vi "Read Scalar Data.vi"(8 "error in (no error)":errorcluster, 10 "Values":dbl[](array[numeric]), 11 "Cluster":T1 {"Data Type" format="%.0x"}) -> (0 "error out":errorcluster, 2 "Values":dbl[](array[numeric]), 3 "Cluster":T1 {"Data Type" format="%.0x"})   [LabVIEW 2016, in "FPGA Addon Engine.lvlib"]
uses:
  FPGA Addon Engine.lvlib
  Types/Register Settings.ctl
  FPGA-Resource-Manager-APIs/Source/Shared/Types/Data Type.ctl
  FPGA-Resource-Manager-APIs/Source/Shared/Types/Scalar Type.ctl
  <vilib>/rvi/errors/niLvFpgaAdjustHostInterfaceError.vi
  <vilib>/Utility/error.llb/Error Cluster From Error Code.vi
  <vilib>/rvi/interface/nirviReadWriteControl/nirviReadWriteControl.xnode
  NiFpgaLv.dll
  <vilib>/rvi/interface/Simulation/niFpgaSimulationCallBeginRW.vi
  FPGA-Resource-Manager-APIs/Source/Shared/FPGA RM Shared API.lvlib
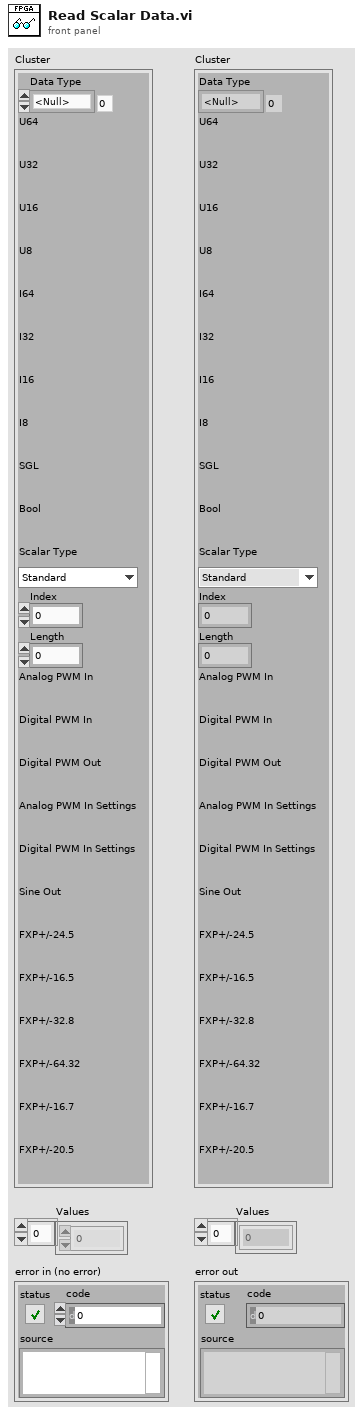
[diagram p1: front panel]
types:
  T1 = typedef "FPGA Addon Engine.lvlib/Register Settings.ctl" = cluster{"Data Type":T2, "U64":refnum<k20>, "U32":refnum<k20>, "U16":refnum<k20>, "U8":refnum<k20>, "I64":refnum<k20>, "I32":refnum<k20>, "I16":refnum<k20>, "I8":refnum<k20>, "SGL":refnum<k20>, "Bool":refnum<k20>, "Scalar Type":T3, "Index":i32, "Length":i32, "Analog PWM In":refnum<k20>, "Digital PWM In":refnum<k20>, "Digital PWM Out":refnum<k20>, "Analog PWM In Settings":refnum<k20>, "Digital PWM In Settings":refnum<k20>, "Sine Out":refnum<k20>, "FXP+/-24.5":refnum<k20>, "FXP+/-16.5":refnum<k20>, "FXP+/-32.8":refnum<k20>, "FXP+/-64.32":refnum<k20>, "FXP+/-16.7":refnum<k20>, "FXP+/-20.5":refnum<k20>}
  T2 = typedef "FPGA RM Shared API.lvlib/Data Type.ctl" = enum8{"<Null>", "I8", "I16", "I32", "I64", "U8", "U16", "U32", "U64", "SGL", "Boolean", "Analog PWM In Settings", "Analog PWM In", "Digital PWM In Settings", "Digital PWM In", "Digital PWM Out", "Sine Out", "FXP+/-24.5", "FXP+/-16.5", "FXP+/-32.8", "FXP+/-64.32", "FXP+/-16.7", "FXP+/-20.5"}
  T3 = typedef "FPGA RM Shared API.lvlib/Scalar Type.ctl" = enum16{"Standard", "Bitpacked"}
  T4 = cluster{"ACTIVE TICKS":u32, "INACTIVE TICKS":u32, "ACQ TICKS":u32, "ACTIVE VOLTAGE":fxp<+/-,32,8>, "INACTIVE VOLTAGE":fxp<+/-,32,8>}
  T5 = cluster{"ACTIVE TICKS":u32, "INACTIVE TICKS":u32, "ACQ TICKS":u32}
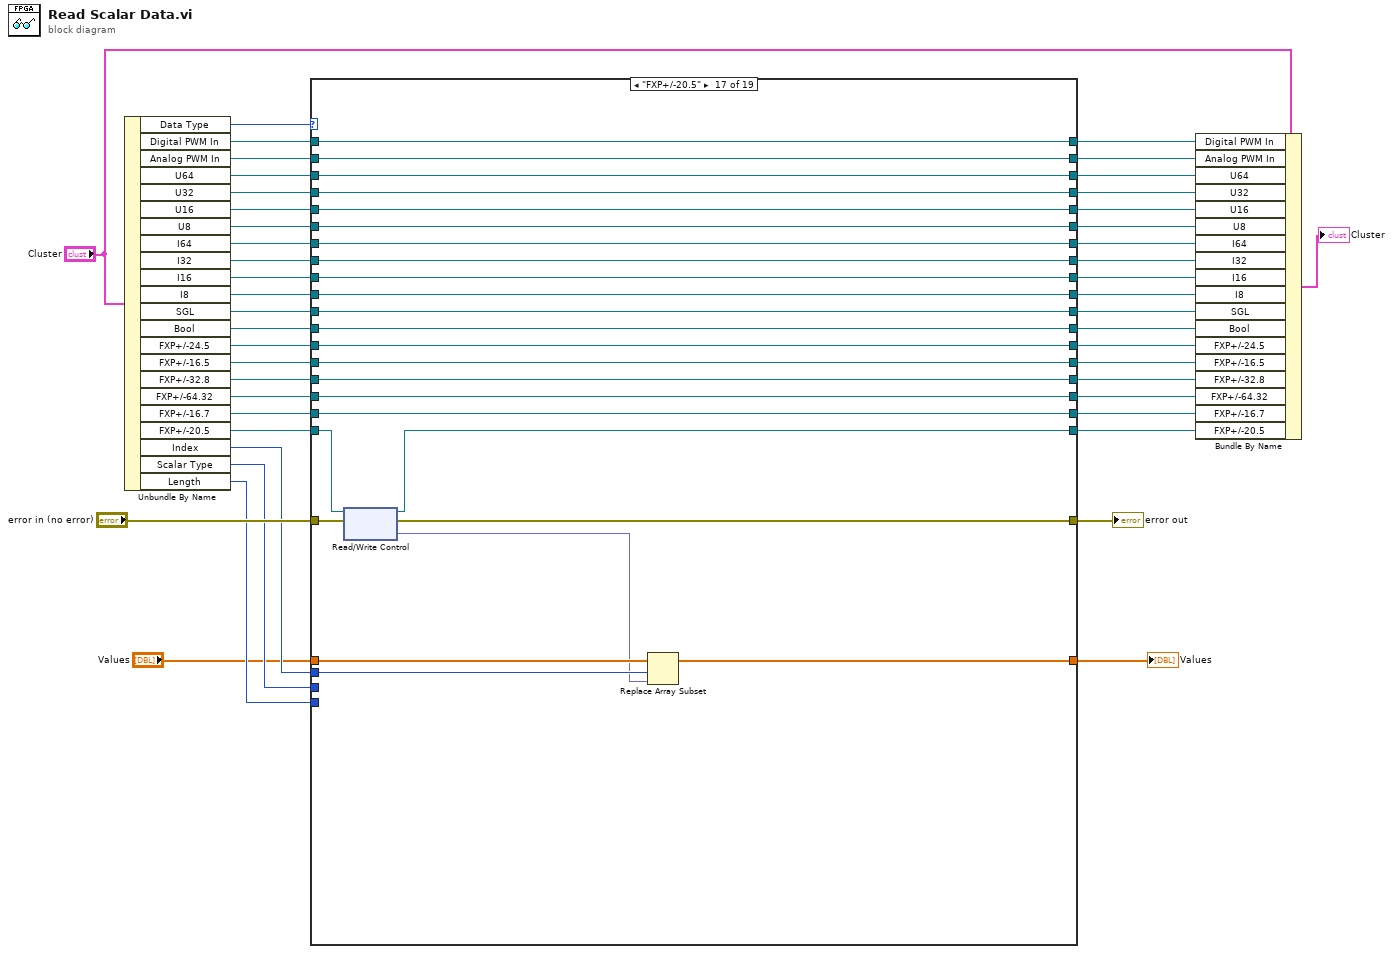
[diagram p0: block diagram]
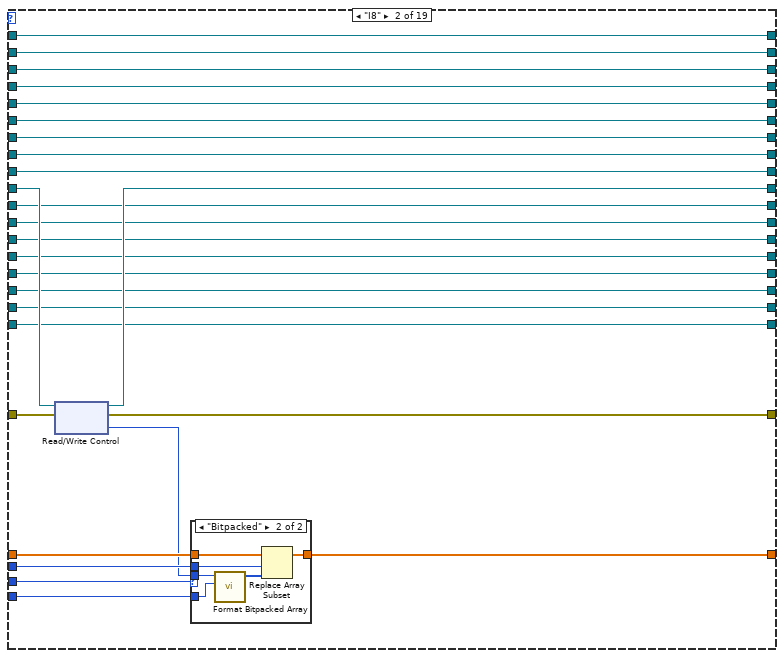
[diagram p3: hidden frame]
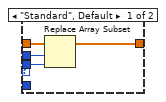
[diagram p4: hidden frame]
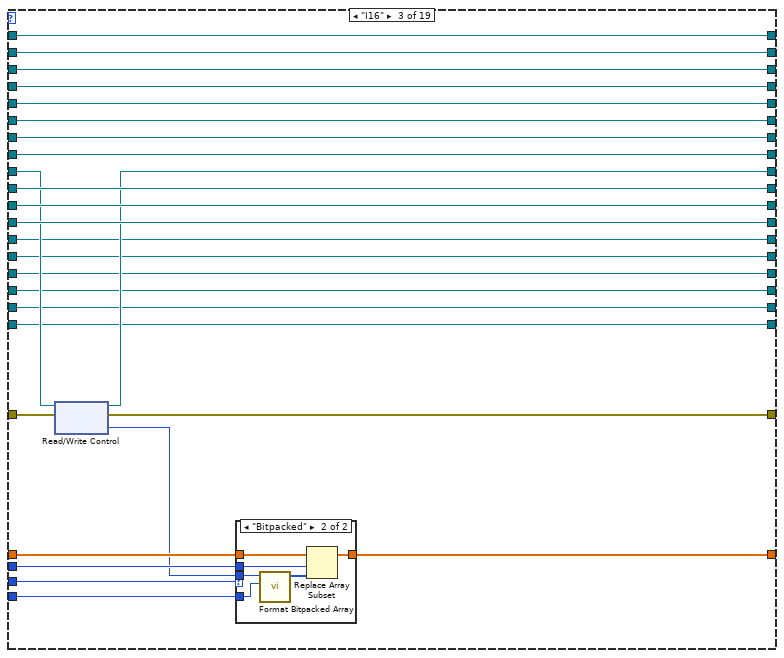
[diagram p5: hidden frame]
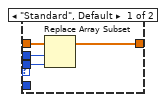
[diagram p6: hidden frame]
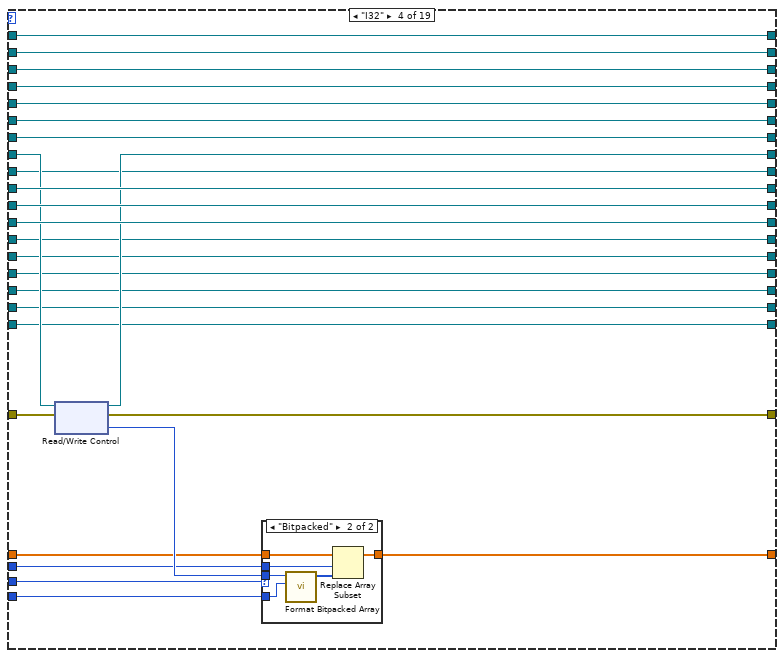
[diagram p7: hidden frame]
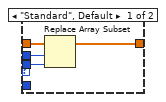
[diagram p8: hidden frame]
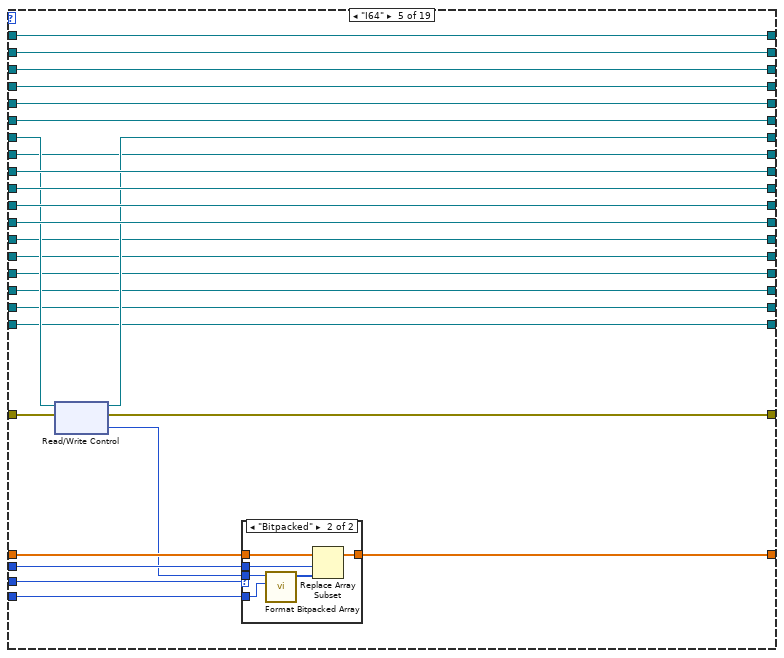
[diagram p9: hidden frame]
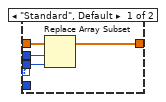
[diagram p10: hidden frame]
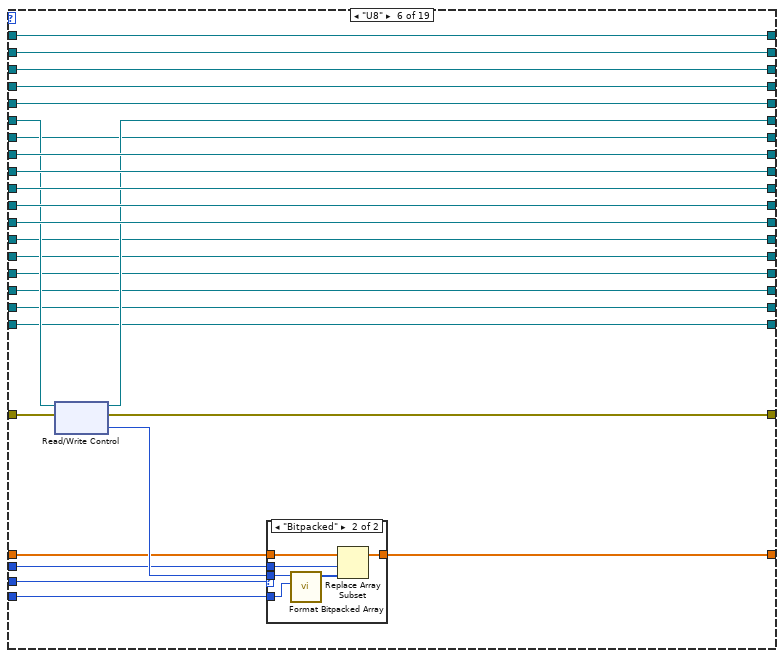
[diagram p11: hidden frame]
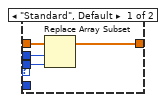
[diagram p12: hidden frame]
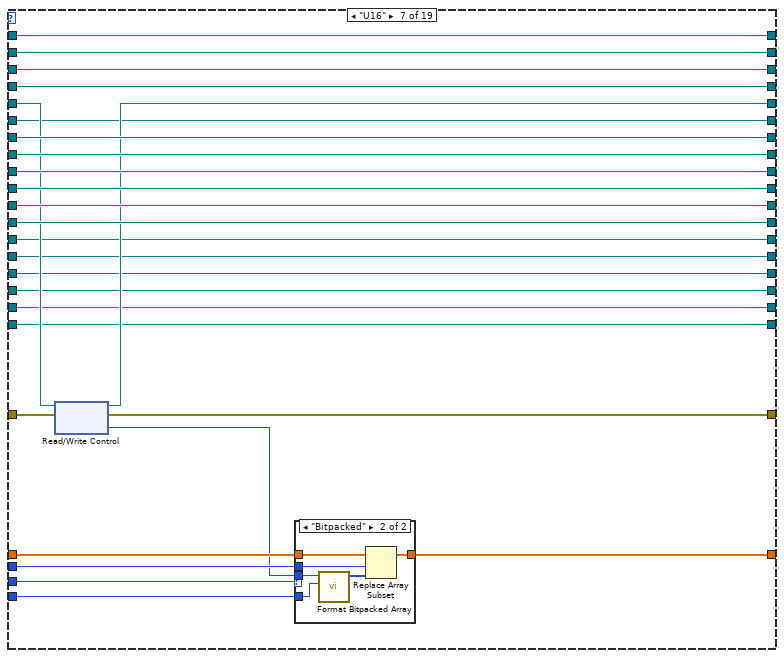
[diagram p13: hidden frame]
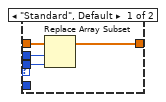
[diagram p14: hidden frame]
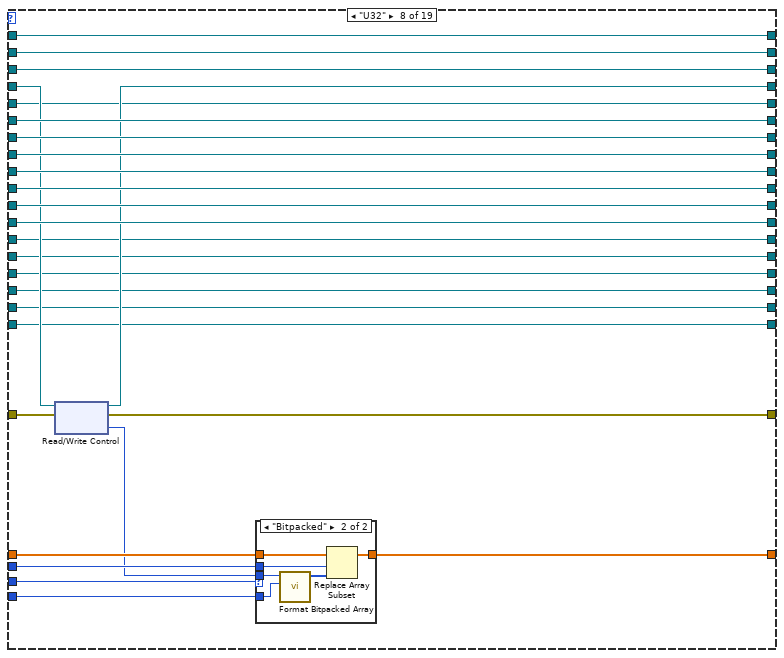
[diagram p15: hidden frame]
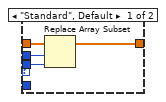
[diagram p16: hidden frame]
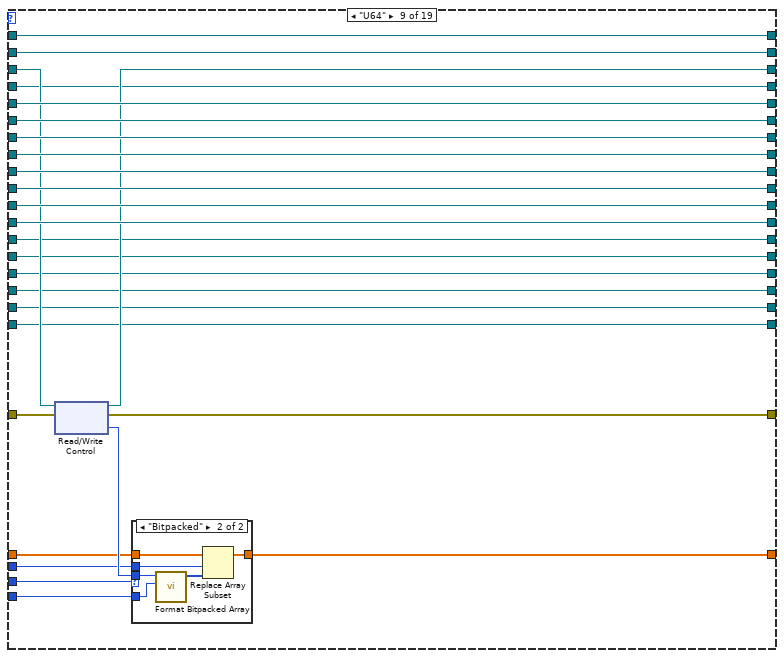
[diagram p17: hidden frame]
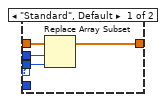
[diagram p18: hidden frame]
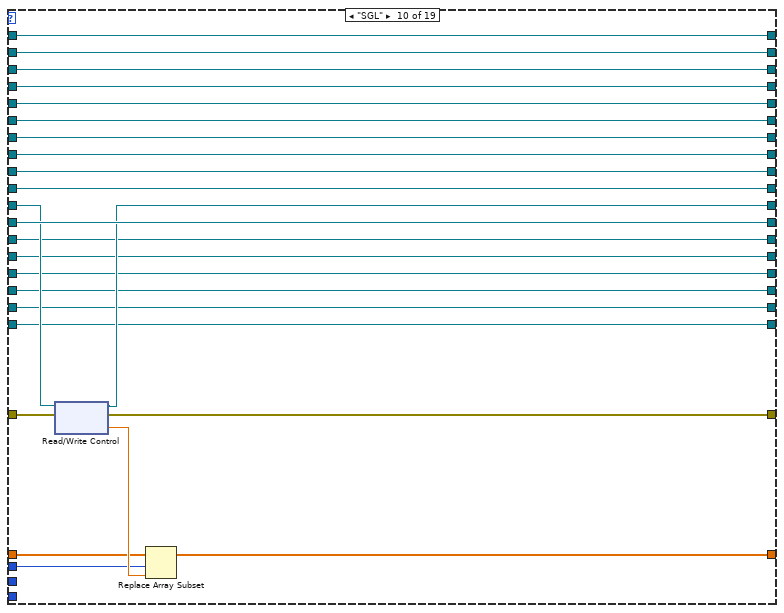
[diagram p19: hidden frame]
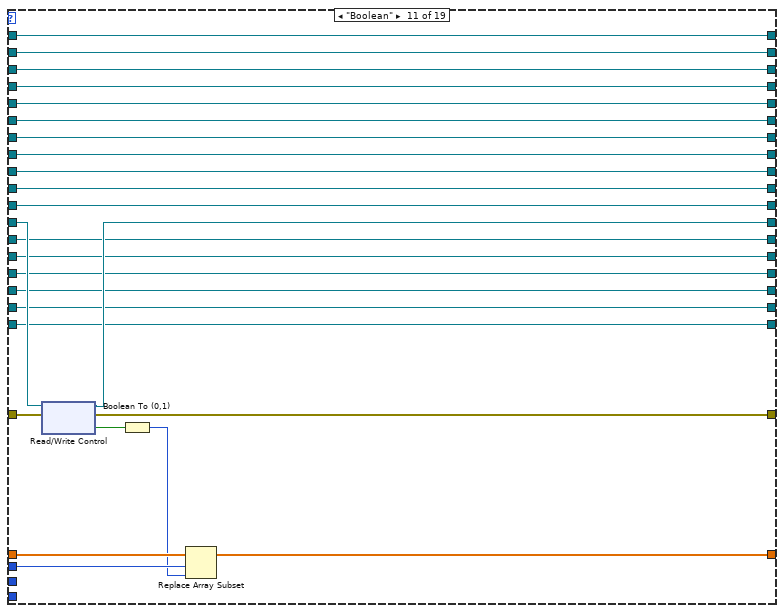
[diagram p20: hidden frame]
diagram:
  n1 = Unbundle By Name("Cluster") -> ("Data Type"=w46:T2, "Digital PWM In"=w14:refnum<k20>, "Analog PWM In"=w15:refnum<k20>, "U64"=w23:refnum<k20>, "U32"=w25:refnum<k20>, "U16"=w27:refnum<k20>, "U8"=w29:refnum<k20>, "I64"=w31:refnum<k20>, "I32"=w33:refnum<k20>, "I16"=w35:refnum<k20>, "I8"=w45:refnum<k20>, "SGL"=w39:refnum<k20>, "Bool"=w38:refnum<k20>, "FXP+/-24.5"=w12:refnum<k20>, "FXP+/-16.5"=w9:refnum<k20>, "FXP+/-32.8"=w8:refnum<k20>, "FXP+/-64.32"=w5:refnum<k20>, "FXP+/-16.7"=w3:refnum<k20>, "FXP+/-20.5"=w1:refnum<k20>, "Index"=w19:i32, "Scalar Type"=w20:T3, "Length"=w21:i32)
  n2 = case shown="\"FXP+/-20.5\"" w46 {
    tunnel: w45 -> [w64 w93 w120 w158 w196 w234 w272 w310 w348 w384 w411 w436 w461 w486 w511 w536 w561 w601 w651]
    tunnel: "error in (no error)" -> [w56 w92 w130 w167 w204 w241 w278 w315 w352 w387 w413 w438 w463 w488 w513 w538 w563 w598 w648]
    tunnel: [w56 w91 w129 w166 w203 w240 w277 w314 w351 w386 w412 w437 w462 w487 w512 w537 w562 w597 w647] -> w43
    tunnel: [w64 w90 w120 w158 w196 w234 w272 w310 w348 w384 w411 w436 w461 w486 w511 w536 w561 w601 w651] -> w41
    tunnel: [w65 w89 w128 w165 w202 w239 w276 w313 w350 w375 w401 w428 w453 w478 w503 w528 w553 w600 w650] -> w40
    tunnel: w39 -> [w65 w89 w128 w165 w202 w239 w276 w313 w350 w377 w401 w428 w453 w478 w503 w528 w553 w600 w650]
    tunnel: w38 -> [w66 w88 w127 w164 w201 w238 w275 w312 w349 w385 w403 w421 w447 w472 w497 w522 w547 w599 w649]
    tunnel: [w66 w88 w127 w164 w201 w238 w275 w312 w349 w385 w402 w421 w447 w472 w497 w522 w547 w599 w649] -> w37
    tunnel: [w63 w87 w118 w155 w195 w233 w271 w309 w347 w383 w410 w435 w460 w485 w510 w535 w560 w602 w652] -> w36
    tunnel: w35 -> [w63 w87 w119 w155 w195 w233 w271 w309 w347 w383 w410 w435 w460 w485 w510 w535 w560 w602 w652]
    tunnel: [w62 w86 w126 w156 w192 w232 w270 w308 w346 w382 w409 w434 w459 w484 w509 w534 w559 w603 w653] -> w34
    tunnel: w33 -> [w62 w86 w126 w157 w192 w232 w270 w308 w346 w382 w409 w434 w459 w484 w509 w534 w559 w603 w653]
    tunnel: [w61 w85 w125 w163 w193 w229 w269 w307 w345 w381 w408 w433 w458 w483 w508 w533 w558 w604 w654] -> w32
    tunnel: w31 -> [w61 w85 w125 w163 w194 w229 w269 w307 w345 w381 w408 w433 w458 w483 w508 w533 w558 w604 w654]
    tunnel: [w60 w84 w124 w162 w200 w230 w266 w306 w344 w380 w407 w432 w457 w482 w507 w532 w557 w605 w655] -> w30
    tunnel: w29 -> [w60 w84 w124 w162 w200 w231 w266 w306 w344 w380 w407 w432 w457 w482 w507 w532 w557 w605 w655]
    tunnel: [w59 w83 w123 w161 w199 w237 w267 w303 w343 w379 w406 w431 w456 w481 w506 w531 w556 w606 w656] -> w28
    tunnel: w27 -> [w59 w83 w123 w161 w199 w237 w268 w303 w343 w379 w406 w431 w456 w481 w506 w531 w556 w606 w656]
    tunnel: [w58 w82 w122 w160 w198 w236 w274 w304 w340 w378 w405 w430 w455 w480 w505 w530 w555 w607 w657] -> w26
    tunnel: w25 -> [w58 w82 w122 w160 w198 w236 w274 w305 w340 w378 w405 w430 w455 w480 w505 w530 w555 w607 w657]
    tunnel: [w57 w81 w121 w159 w197 w235 w273 w311 w341 w376 w404 w429 w454 w479 w504 w529 w554 w608 w658] -> w24
    tunnel: w23 -> [w57 w81 w121 w159 w197 w235 w273 w311 w342 w376 w404 w429 w454 w479 w504 w529 w554 w608 w658]
    tunnel: w21 -> [_ w77 w114 w149 w188 w225 w265 w298 w336 _ _ _ _ _ _ _ _ _ _]
    tunnel: w20 -> [_ w78 w115 w150 w189 w224 w264 w299 w337 _ _ _ _ _ _ _ _ _ _]
    tunnel: w19 -> [_ w79 w116 w153 w190 w226 w263 w300 w338 w373 w399 w427 w452 w477 w502 w527 w552 w580 w630]
    tunnel: "Values" -> [w55 w80 w117 w152 w191 w227 w262 w302 w335 w372 w398 w426 w451 w476 w501 w526 w551 w582 w632]
    tunnel: [w55 w75 w112 w151 w186 w223 w261 w301 w334 w371 w396 w425 w450 w475 w500 w525 w550 w581 w631] -> w17
    tunnel: [w54 w73 w110 w147 w184 w221 w258 w295 w332 w369 w394 w423 w448 w473 w498 w523 w548 w595 w628] -> w16
    tunnel: w15 -> [w54 w73 w110 w147 w184 w221 w258 w295 w332 w369 w394 w423 w448 w473 w498 w523 w548 w596 w628]
    tunnel: w14 -> [w53 w74 w111 w148 w185 w222 w259 w296 w333 w370 w395 w424 w449 w474 w499 w524 w549 w609 w627]
    tunnel: [w53 w74 w111 w148 w185 w222 w259 w296 w333 w370 w395 w424 w449 w474 w499 w524 w549 w609 w626] -> w13
    tunnel: w12 -> [w52 w72 w109 w146 w183 w220 w257 w294 w331 w368 w393 w422 w441 w469 w495 w520 w545 w569 w620]
    tunnel: [w52 w72 w109 w146 w183 w220 w257 w294 w331 w368 w393 w420 w441 w469 w495 w520 w545 w569 w620] -> w11
    tunnel: [w51 w71 w108 w145 w182 w219 w256 w293 w330 w367 w392 w418 w442 w468 w494 w519 w544 w568 w619] -> w10
    tunnel: w9 -> [w51 w71 w108 w145 w182 w219 w256 w293 w330 w367 w392 w418 w443 w468 w494 w519 w544 w568 w619]
    tunnel: w8 -> [w50 w70 w107 w144 w181 w218 w255 w292 w329 w366 w391 w417 w445 w467 w493 w518 w543 w567 w618]
    tunnel: [w50 w70 w107 w144 w181 w218 w255 w292 w329 w366 w391 w417 w445 w466 w493 w518 w543 w567 w618] -> w7
    tunnel: [w49 w69 w106 w143 w180 w217 w254 w291 w328 w365 w390 w416 w444 w470 w491 w517 w542 w566 w617] -> w6
    tunnel: w5 -> [w49 w69 w106 w143 w180 w217 w254 w291 w328 w365 w390 w416 w444 w470 w492 w517 w542 w566 w617]
    tunnel: [w48 w68 w105 w142 w179 w216 w253 w290 w327 w364 w389 w415 w440 w465 w490 w515 w539 w565 w616] -> w4
    tunnel: w3 -> [w48 w68 w105 w142 w179 w216 w253 w290 w327 w364 w389 w415 w440 w465 w490 w516 w539 w565 w616]
    tunnel: [w47 w67 w104 w141 w178 w215 w252 w289 w326 w363 w388 w414 w439 w464 w489 w514 w541 w564 w615] -> w2
    tunnel: w1 -> [w47 w67 w104 w141 w178 w215 w252 w289 w326 w363 w388 w414 w439 w464 w489 w514 w540 w564 w615]
    frame "<Null>", Default {
    }
    frame "I8" {
      n3 = xnode "Read/Write Control"("FPGA VI Reference In"=w93, "error in"=w92) -> ("FPGA VI Reference Out"=w90:refnum<k20>, "error out"=w91:errorcluster, "Value"=w76:i8)
      n4 = case shown="\"Bitpacked\"" w78 {
        tunnel: w80 -> [w97 w101]
        tunnel: [w96 w100] -> w75
        tunnel: w76 -> [w95 w103]
        tunnel: w79 -> [w94 w98]
        tunnel: w77 -> [_ w102]
        frame "Standard", Default {
          n5 = Replace Array Subset(array=w97, new element=w95, index=w94) -> (w96:dbl[])
        }
        frame "Bitpacked" {
          n6 = call "Format Bitpacked Array.vi"("Length"=w102, "Value"=w103) -> ("Array"=w99:i16[])  [unwired: 9 in]
          n7 = Replace Array Subset(array=w101, new element=w99, index=w98) -> (w100:dbl[])
        }
      }
    }
    frame "I16" {
      n8 = xnode "Read/Write Control"("FPGA VI Reference In"=w119, "error in"=w130) -> ("FPGA VI Reference Out"=w118:refnum<k20>, "error out"=w129:errorcluster, "Value"=w113:i16)
      n9 = case shown="\"Bitpacked\"" w115 {
        tunnel: w117 -> [w134 w138]
        tunnel: [w133 w137] -> w112
        tunnel: w113 -> [w132 w140]
        tunnel: w116 -> [w131 w135]
        tunnel: w114 -> [_ w139]
        frame "Standard", Default {
          n10 = Replace Array Subset(array=w134, new element=w132, index=w131) -> (w133:dbl[])
        }
        frame "Bitpacked" {
          n11 = call "Format Bitpacked Array.vi"("Length"=w139, "Value"=w140) -> ("Array"=w136:i16[])  [unwired: 9 in]
          n12 = Replace Array Subset(array=w138, new element=w136, index=w135) -> (w137:dbl[])
        }
      }
    }
    frame "I32" {
      n13 = xnode "Read/Write Control"("FPGA VI Reference In"=w157, "error in"=w167) -> ("FPGA VI Reference Out"=w156:refnum<k20>, "error out"=w166:errorcluster, "Value"=w154:i32)
      n14 = case shown="\"Bitpacked\"" w150 {
        tunnel: w152 -> [w171 w175]
        tunnel: [w170 w174] -> w151
        tunnel: w154 -> [w169 w177]
        tunnel: w153 -> [w168 w172]
        tunnel: w149 -> [_ w176]
        frame "Standard", Default {
          n15 = Replace Array Subset(array=w171, new element=w169, index=w168) -> (w170:dbl[])
        }
        frame "Bitpacked" {
          n16 = call "Format Bitpacked Array.vi"("Length"=w176, "Value"=w177) -> ("Array"=w173:i16[])  [unwired: 9 in]
          n17 = Replace Array Subset(array=w175, new element=w173, index=w172) -> (w174:dbl[])
        }
      }
    }
    frame "I64" {
      n18 = xnode "Read/Write Control"("FPGA VI Reference In"=w194, "error in"=w204) -> ("FPGA VI Reference Out"=w193:refnum<k20>, "error out"=w203:errorcluster, "Value"=w187:i64)
      n19 = case shown="\"Bitpacked\"" w189 {
        tunnel: w191 -> [w208 w212]
        tunnel: [w207 w211] -> w186
        tunnel: w187 -> [w206 w214]
        tunnel: w190 -> [w205 w209]
        tunnel: w188 -> [_ w213]
        frame "Standard", Default {
          n20 = Replace Array Subset(array=w208, new element=w206, index=w205) -> (w207:dbl[])
        }
        frame "Bitpacked" {
          n21 = call "Format Bitpacked Array.vi"("Length"=w213, "Value"=w214) -> ("Array"=w210:i16[])  [unwired: 9 in]
          n22 = Replace Array Subset(array=w212, new element=w210, index=w209) -> (w211:dbl[])
        }
      }
    }
    frame "U8" {
      n23 = xnode "Read/Write Control"("FPGA VI Reference In"=w231, "error in"=w241) -> ("FPGA VI Reference Out"=w230:refnum<k20>, "error out"=w240:errorcluster, "Value"=w228:u8)
      n24 = case shown="\"Bitpacked\"" w224 {
        tunnel: w227 -> [w245 w249]
        tunnel: [w244 w248] -> w223
        tunnel: w228 -> [w243 w251]
        tunnel: w226 -> [w242 w246]
        tunnel: w225 -> [_ w250]
        frame "Standard", Default {
          n25 = Replace Array Subset(array=w245, new element=w243, index=w242) -> (w244:dbl[])
        }
        frame "Bitpacked" {
          n26 = call "Format Bitpacked Array.vi"("Length"=w250, "Value"=w251) -> ("Array"=w247:i16[])  [unwired: 9 in]
          n27 = Replace Array Subset(array=w249, new element=w247, index=w246) -> (w248:dbl[])
        }
      }
    }
    frame "U16" {
      n28 = xnode "Read/Write Control"("FPGA VI Reference In"=w268, "error in"=w278) -> ("FPGA VI Reference Out"=w267:refnum<k20>, "error out"=w277:errorcluster, "Value"=w260:u16)
      n29 = case shown="\"Bitpacked\"" w264 {
        tunnel: w262 -> [w282 w286]
        tunnel: [w281 w285] -> w261
        tunnel: w260 -> [w280 w288]
        tunnel: w263 -> [w279 w283]
        tunnel: w265 -> [_ w287]
        frame "Standard", Default {
          n30 = Replace Array Subset(array=w282, new element=w280, index=w279) -> (w281:dbl[])
        }
        frame "Bitpacked" {
          n31 = call "Format Bitpacked Array.vi"("Length"=w287, "Value"=w288) -> ("Array"=w284:i16[])  [unwired: 9 in]
          n32 = Replace Array Subset(array=w286, new element=w284, index=w283) -> (w285:dbl[])
        }
      }
    }
    frame "U32" {
      n33 = xnode "Read/Write Control"("FPGA VI Reference In"=w305, "error in"=w315) -> ("FPGA VI Reference Out"=w304:refnum<k20>, "error out"=w314:errorcluster, "Value"=w297:u32)
      n34 = case shown="\"Bitpacked\"" w299 {
        tunnel: w302 -> [w319 w323]
        tunnel: [w318 w322] -> w301
        tunnel: w297 -> [w317 w325]
        tunnel: w300 -> [w316 w320]
        tunnel: w298 -> [_ w324]
        frame "Standard", Default {
          n35 = Replace Array Subset(array=w319, new element=w317, index=w316) -> (w318:dbl[])
        }
        frame "Bitpacked" {
          n36 = call "Format Bitpacked Array.vi"("Length"=w324, "Value"=w325) -> ("Array"=w321:i16[])  [unwired: 9 in]
          n37 = Replace Array Subset(array=w323, new element=w321, index=w320) -> (w322:dbl[])
        }
      }
    }
    frame "U64" {
      n38 = xnode "Read/Write Control"("FPGA VI Reference In"=w342, "error in"=w352) -> ("FPGA VI Reference Out"=w341:refnum<k20>, "error out"=w351:errorcluster, "Value"=w339:u64)
      n39 = case shown="\"Bitpacked\"" w337 {
        tunnel: w335 -> [w356 w360]
        tunnel: [w355 w359] -> w334
        tunnel: w339 -> [w354 w362]
        tunnel: w338 -> [w353 w357]
        tunnel: w336 -> [_ w361]
        frame "Standard", Default {
          n40 = Replace Array Subset(array=w356, new element=w354, index=w353) -> (w355:dbl[])
        }
        frame "Bitpacked" {
          n41 = call "Format Bitpacked Array.vi"("Length"=w361, "Value"=w362) -> ("Array"=w358:i16[])  [unwired: 9 in]
          n42 = Replace Array Subset(array=w360, new element=w358, index=w357) -> (w359:dbl[])
        }
      }
    }
    frame "SGL" {
      n43 = xnode "Read/Write Control"("FPGA VI Reference In"=w377, "error in"=w387) -> ("FPGA VI Reference Out"=w375:refnum<k20>, "error out"=w386:errorcluster, "Value"=w374:sgl)
      n44 = Replace Array Subset(array=w372, new element=w374, index=w373) -> (w371:dbl[])
    }
    frame "Boolean" {
      n45 = xnode "Read/Write Control"("FPGA VI Reference In"=w403, "error in"=w413) -> ("FPGA VI Reference Out"=w402:refnum<k20>, "error out"=w412:errorcluster, "Value"=w400:bool)
      n46 = Boolean To (0,1)(Boolean=w400) -> (0, 1=w397:i16)
      n47 = Replace Array Subset(array=w398, new element=w397, index=w399) -> (w396:dbl[])
    }
    frame "FXP+/-24.5" {
      n48 = xnode "Read/Write Control"("FPGA VI Reference In"=w422, "error in"=w438) -> ("FPGA VI Reference Out"=w420:refnum<k20>, "error out"=w437:errorcluster, "Value"=w419:fxp<+/-,24,5>)
      n49 = Replace Array Subset(array=w426, new element=w419, index=w427) -> (w425:dbl[])
    }
    frame "FXP+/-16.5" {
      n50 = xnode "Read/Write Control"("FPGA VI Reference In"=w443, "error in"=w463) -> ("FPGA VI Reference Out"=w442:refnum<k20>, "error out"=w462:errorcluster, "Value"=w446:fxp<+/-,16,5>)
      n51 = Replace Array Subset(array=w451, new element=w446, index=w452) -> (w450:dbl[])
    }
    frame "FXP+/-32.8" {
      n52 = xnode "Read/Write Control"("FPGA VI Reference In"=w467, "error in"=w488) -> ("FPGA VI Reference Out"=w466:refnum<k20>, "error out"=w487:errorcluster, "Value"=w471:fxp<+/-,32,8>)
      n53 = Replace Array Subset(array=w476, new element=w471, index=w477) -> (w475:dbl[])
    }
    frame "FXP+/-64.32" {
      n54 = xnode "Read/Write Control"("FPGA VI Reference In"=w492, "error in"=w513) -> ("FPGA VI Reference Out"=w491:refnum<k20>, "error out"=w512:errorcluster, "Value"=w496:fxp<+/-,64,32>)
      n55 = Replace Array Subset(array=w501, new element=w496, index=w502) -> (w500:dbl[])
    }
    frame "FXP+/-16.7" {
      n56 = xnode "Read/Write Control"("FPGA VI Reference In"=w516, "error in"=w538) -> ("FPGA VI Reference Out"=w515:refnum<k20>, "error out"=w537:errorcluster, "Value"=w521:fxp<+/-,16,7>)
      n57 = Replace Array Subset(array=w526, new element=w521, index=w527) -> (w525:dbl[])
    }
    frame "FXP+/-20.5" {
      n58 = xnode "Read/Write Control"("FPGA VI Reference In"=w540, "error in"=w563) -> ("FPGA VI Reference Out"=w541:refnum<k20>, "error out"=w562:errorcluster, "Value"=w546:fxp<+/-,20,5>)
      n59 = Replace Array Subset(array=w551, new element=w546, index=w552) -> (w550:dbl[])
    }
    frame "Analog PWM In" {
      w589 = 2.5000000292152436e-08 ("y")
      n60 = xnode "Read/Write Control"("FPGA VI Reference In"=w596, "error in"=w598) -> ("FPGA VI Reference Out"=w595:refnum<k20>, "error out"=w597:errorcluster, "Value"=w577:T4)
      n61 = Unbundle By Name(w577) -> ("ACTIVE TICKS"=w576:u32, "INACTIVE TICKS"=w575:u32, "ACQ TICKS"=w574:u32, "ACTIVE VOLTAGE"=w573:fxp<+/-,32,8>, "INACTIVE VOLTAGE"=w572:fxp<+/-,32,8>)
      n62 = Add(x=w576, y=w575) -> (x+y=w591:u32)
      n63 = Compound Arithmetic op=MULTIPLY(w591, w574, w589) -> (w592:dbl)
      n64 = Divide(x=w576, y=w591) -> (x/y=w585:dbl)
      n65 = Compound Arithmetic op=MULTIPLY(w576, w574, w589) -> (w590:dbl)
      n66 = Multiply(x=100.0, y=w585) -> (x*y=w584:dbl)
      n67 = Equal?(x=0.0, y=w592) -> (x = y?=w588:bool)
      n68 = Reciprocal(x=w592) -> (1/x=w593:dbl)
      n69 = case shown="False" w588 {
        tunnel: [w610 w614] -> w571
        tunnel: [w611 w614] -> w578
        tunnel: [w613 w614] -> w570
        tunnel: w592 -> [w613 _]
        tunnel: [w612 w614] -> w583
        tunnel: w590 -> [w612 _]
        tunnel: w584 -> [w611 _]
        tunnel: w593 -> [w610 _]
        tunnel: 0.0 ("x") -> [_ w614]
        frame False {
        }
        frame True {
        }
      }
      n70 = Build Array(w571, w570, w578, w583, w573, w572) -> (w579:dbl[])
      n71 = Replace Array Subset(array=w582, new element=w579, index=w580) -> (w581:dbl[])
    }
    frame "Digital PWM In" {
      w641 = 2.5000000292152436e-08 ("y")
      n72 = xnode "Read/Write Control"("FPGA VI Reference In"=w627, "error in"=w648) -> ("FPGA VI Reference Out"=w626:refnum<k20>, "error out"=w647:errorcluster, "Value"=w634:T5)
      n73 = Unbundle By Name(w634) -> ("ACTIVE TICKS"=w624:u32, "INACTIVE TICKS"=w623:u32, "ACQ TICKS"=w637:u32)
      n74 = Add(x=w624, y=w623) -> (x+y=w643:u32)
      n75 = Compound Arithmetic op=MULTIPLY(w643, w637, w641) -> (w644:dbl)
      n76 = Divide(x=w624, y=w643) -> (x/y=w636:dbl)
      n77 = Compound Arithmetic op=MULTIPLY(w624, w637, w641) -> (w642:dbl)
      n78 = Multiply(x=100.0, y=w636) -> (x*y=w635:dbl)
      n79 = Equal?(x=0.0, y=w644) -> (x = y?=w640:bool)
      n80 = Reciprocal(x=w644) -> (1/x=w645:dbl)
      n81 = case shown="False" w640 {
        tunnel: [w659 w663] -> w622
        tunnel: [w660 w663] -> w625
        tunnel: [w662 w663] -> w621
        tunnel: w644 -> [w662 _]
        tunnel: [w661 w663] -> w633
        tunnel: w642 -> [w661 _]
        tunnel: w635 -> [w660 _]
        tunnel: w645 -> [w659 _]
        tunnel: 0.0 ("x") -> [_ w663]
        frame False {
        }
        frame True {
        }
      }
      n82 = Build Array(w622, w621, w625, w633) -> (w629:dbl[])
      n83 = Replace Array Subset(array=w632, new element=w629, index=w630) -> (w631:dbl[])
    }
  }
  "error out" <- w43
  "Values" <- w17
  n84 = Bundle By Name(cluster="Cluster", "Digital PWM In"=w13, "Analog PWM In"=w16, "U64"=w24, "U32"=w26, "U16"=w28, "U8"=w30, "I64"=w32, "I32"=w34, "I16"=w36, "I8"=w41, "SGL"=w40, "Bool"=w37, "FXP+/-24.5"=w11, "FXP+/-16.5"=w10, "FXP+/-32.8"=w7, "FXP+/-64.32"=w6, "FXP+/-16.7"=w4, "FXP+/-20.5"=w2) -> (→"Cluster":T1)
